vi "Default Broadcast (Cloneable)--template.vi"(8 "error in (no error)":errorcluster) -> (0 "error out":errorcluster, 1 "Update Module Execution Status":refnum<user-event>, 2 "Error Reported":refnum<user-event>, 3 "Status Updated":refnum<user-event>, 4 "System Message":refnum<user-event>, 5 "Module Did Stop":refnum<user-event>)   [LabVIEW 2022 SP3, in "hse-dqmh-dynamicrequesters.lvlib"]
doc: "____\nHAMPEL SOFTWARE ENGINEERING v3.8.0 (2023-12-18 14:41)"
uses:
  hse-dqmh-dynamicrequesters.lvlib
  Stop Argument (Cloneable)--cluster.ctl
  Status Updated Argument (Cloneable)--cluster.ctl
  Error Reported Argument (Cloneable)--cluster.ctl
  Get Module Execution Status Argument (Cloneable)--cluster.ctl
  Controls/System Message Argument--cluster.ctl
  Controls/System Message Source.ctl
  hse-dqmh.lvlib
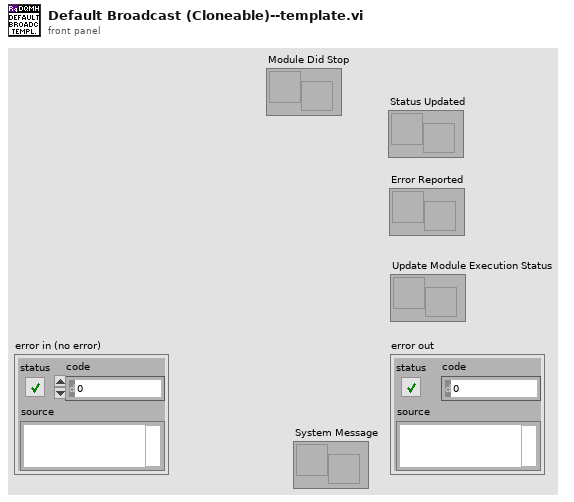
[diagram p1: front panel]
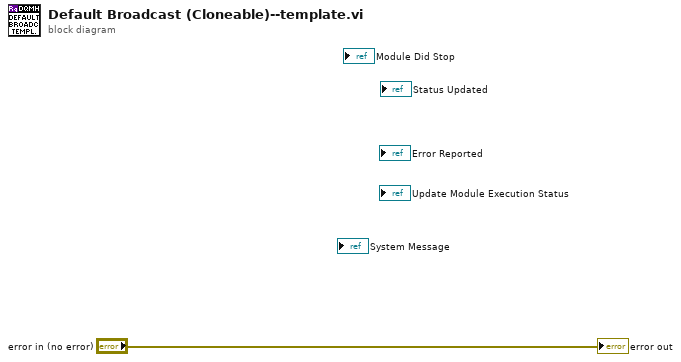
[diagram p0: block diagram]
diagram:
  "error out" <- "error in (no error)"
